vi "Read_instrument.vi"(0 "PrepLinePictureObjects in":refnum<class "PrepLineObject.lvclass">, 3 "error in (no error)":errorcluster) -> (7 "PrepLinePictureObjects out":refnum<class "PrepLineObject.lvclass">, 8 "instrument name":string, 10 "error out":errorcluster)   [LabVIEW 2018, in "PrepLineObject.lvclass"]
doc: "gets the name of the instrument the object interacts with"
uses:
  PrepLineObject.lvclass
  PrepLineObject.lvclass/PrepLineObject.ctl
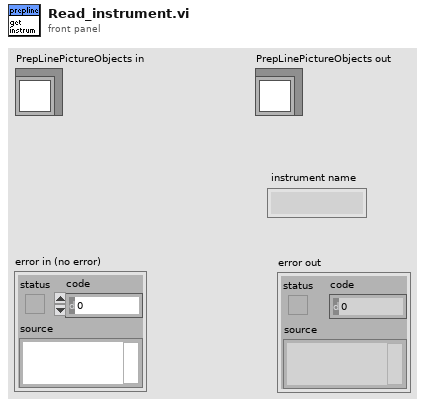
[diagram p1: front panel]
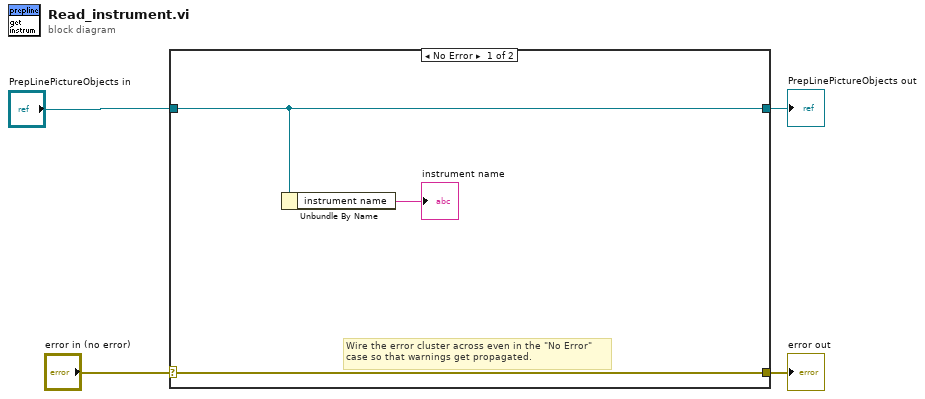
[diagram p0: block diagram]
diagram:
  n1 = case shown="No Error" "error in (no error)" {
    selector: "error in (no error)" -> [w7 w9]
    tunnel: [w7 w9] -> w3
    tunnel: [w5 w8] -> w1
    tunnel: "PrepLinePictureObjects in" -> [w5 w8]
    frame No Error {
      # "Wire the error cluster across even in the \"No Error\"\ncase so that warnings get propagated."
      n2 = Unbundle By Name(w5) -> ("instrument name"=→"instrument name":string)
    }
    frame Error {
    }
  }
  "error out" <- w3
  "PrepLinePictureObjects out" <- w1
